vi "Write then flush.vi"(8 "error in (no error)":errorcluster, 10 "TX Data":string, 11 "Motor_Serial in":refnum<class "Serial.lvclass">) -> (0 "error out":errorcluster, 3 "Motor_Serial out":refnum<class "Serial.lvclass">)   [LabVIEW 2019, in "Serial.lvclass"]
uses:
  Serial.lvclass
  Serial.lvclass/Serial.ctl
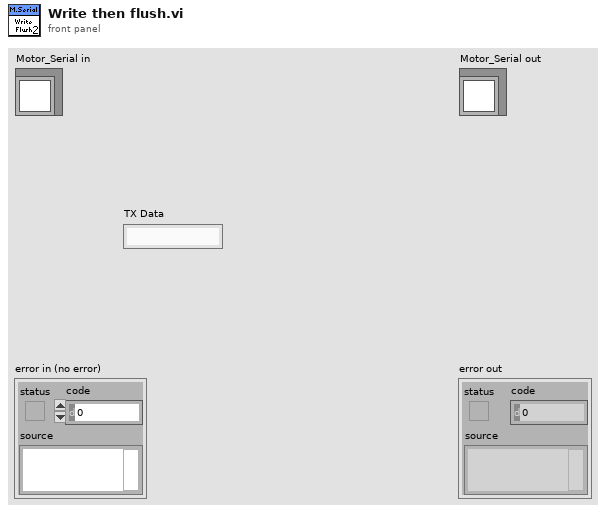
[diagram p1: front panel]
types:
  T1 = typedef "Semaphore RefNum" = refnum<k1>
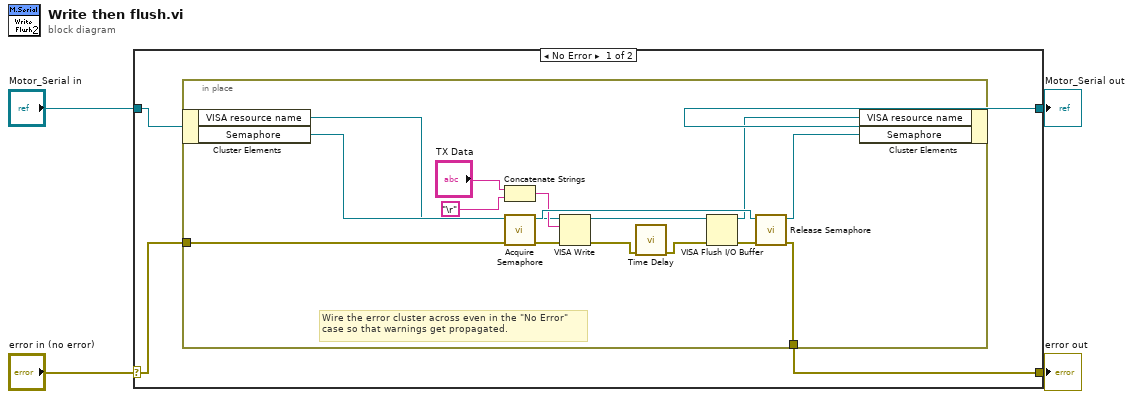
[diagram p0: block diagram]
diagram:
  n1 = case shown="No Error" "error in (no error)" {
    selector: "error in (no error)" -> [w6 w25]
    tunnel: [w7 w24] -> w2
    tunnel: "Motor_Serial in" -> [w8 w24]
    tunnel: [w5 w25] -> w1
    frame No Error {
      n2 = in-place {
        in-place-border: w6 -> [w11]
        in-place-border: [w10] -> w5
        # "Wire the error cluster across even in the \"No Error\"\ncase so that warnings get propagated."
        n3 = in-place-cluster #1(w8) -> ("VISA resource name"=w14:refnum<visa-resource-name>, "Semaphore"=w15:T1)
        n4 = Concatenate Strings("TX Data", "\r") -> (w20:string)
        n5 = call <vilib>:"Acquire Semaphore.vi"("error in (no error)"=w11, "semaphore"=w15) -> ("error out"=w21:errorcluster, "semaphore out"=w22:T1)  [unwired: 3 in, 1 out]
        n6 = VISA Write(VISA resource name=w14, write buffer=w20, error in (no error)=w21) -> (VISA resource name out=w18:refnum<visa-resource-name>, error out=w16:errorcluster)  [unwired: 1 out]
        n7 = call "Time Delay"("error in (no error)"=w16) -> ("error out"=w17:errorcluster)  [unwired: 10 in]
        n8 = VISA Flush I/O Buffer(VISA resource name=w18, error in (no error)=w17) -> (VISA resource name out=w13:refnum<visa-resource-name>, error out=w23:errorcluster)  [unwired: 1 in]
        n9 = call <vilib>:"Release Semaphore.vi"("error in (no error)"=w23, "semaphore"=w22) -> ("error out"=w10:errorcluster, "semaphore out"=w12:T1)  [unwired: 4 in]
        n10 = in-place-cluster #1("VISA resource name"=w13, "Semaphore"=w12) -> (w7:refnum<class "Serial.lvclass">)
      }
    }
    frame Error {
    }
  }
  "error out" <- w1
  "Motor_Serial out" <- w2
